vi "Periodic Tasks.vi"(8 "error in":errorcluster) -> ()   [LabVIEW 2015]
doc: "This VI runs in parallel to other tasks. It can contain as many user-defined periodic loops as you need. These can carry out PID or other sorts of timed response."
uses:
  <vilib>/Rock Robotics/WPI/Solenoid/WPI_SolenoidValue.ctl
  <vilib>/Rock Robotics/WPI/Utilities/WPI_GetSetVariantRefNum.vi
  <vilib>/Rock Robotics/WPI/Solenoid/WPI_SolenoidSetEnum.vi
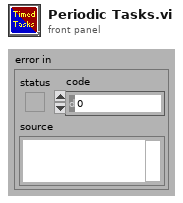
[diagram p1: front panel]
types:
  T1 = typedef "WPI_RobotDriveDevRef.ctl" = cluster{"DevStatus":errorcluster, "Motors[]":T2[], "Square Inputs":bool, "Max Output":dbl}
  T2 = typedef "WPI_MotorControlDeviceRef.ctl" = cluster{"DeviceStatus":errorcluster, "Type":T3, "PWM":cluster{"PWM Channel":T4, "DeadBand":T5}, "CAN":cluster{"Device Number":u8, "Control Mode":T6, "Semaphore":T7, "Max Vout":dbl, "TalonSRX Control Mode":T8}, "Invert":bool}
  T3 = typedef "WPI_MotorControlType.ctl" = enum16{"PWM", "CAN", "CANTalonSRX"}
  T4 = typedef "FPGA_DIOPWMChannel.ctl" = enum8{"PWM 0", "PWM 1", "PWM 2", "PWM 3", "PWM 4", "PWM 5", "PWM 6", "PWM 7", "PWM 8", "PWM 9", "PWM MXP 0", "PWM MXP 1", "PWM MXP 2", "PWM MXP 3", "PWM MXP 4", "PWM MXP 5", "PWM MXP 6", "PWM MXP 7", "PWM MXP 8", "PWM MXP 9", "Invalid"}
  T5 = typedef "WPI_PWMDeadband.ctl" = cluster{"Name":string, "maxPositivePwm":i32, "minPositivePwm":i32, "centerPwm":i32, "maxNegativePwm":i32, "minNegativePwm":i32, "angularRange":u16}
  T6 = typedef "WPI_CANJaguar_ControlMode.ctl" = enum8{"Percent VBus", "Current", "Speed", "Position", "Voltage"}
  T7 = typedef "Semaphore RefNum" = refnum<k1>
  T8 = typedef "WPI_CANTalonSRX_APIControlMode.ctl" = enum8{"Percent VBus", "Speed", "Position", "Slave", "Unchanged / Invalid", "Voltage Compensation", "Current", "Motion Profile"}
  T9 = typedef "WPI_JoystickDevRef.ctl" = cluster{"Device":T10}
  T10 = typedef "WPI_JoystickDeviceEnum.ctl" = enum16{"USB 0", "USB 1", "USB 2", "USB 3", "USB 4", "USB 5"}
  T11 = typedef "WPI_SolenoidDevRef.ctl" = cluster{"DevStatus":errorcluster, "Pneumatics Control Module":u8, "Forward Solenoid Channel":T12, "Reverse Solenoid Channel":T12}
  T12 = typedef "WPI_SolenoidChannel.ctl" = enum8{"Solenoid 0", "Solenoid 1", "Solenoid 2", "Solenoid 3", "Solenoid 4", "Solenoid 5", "Solenoid 6", "Solenoid 7", "Invalid"}
  T13 = cluster{"JoystickDevRef":T9, "RobotDriveDevRef":T1, "SolenoidDevRef":T11, "MotorControlDevRef":T2, "MotorControlDevRef":T2}
  T14 = typedef "WPI_SolenoidValue.ctl" = enum16{"Off", "On", "Forward", "Reverse"}
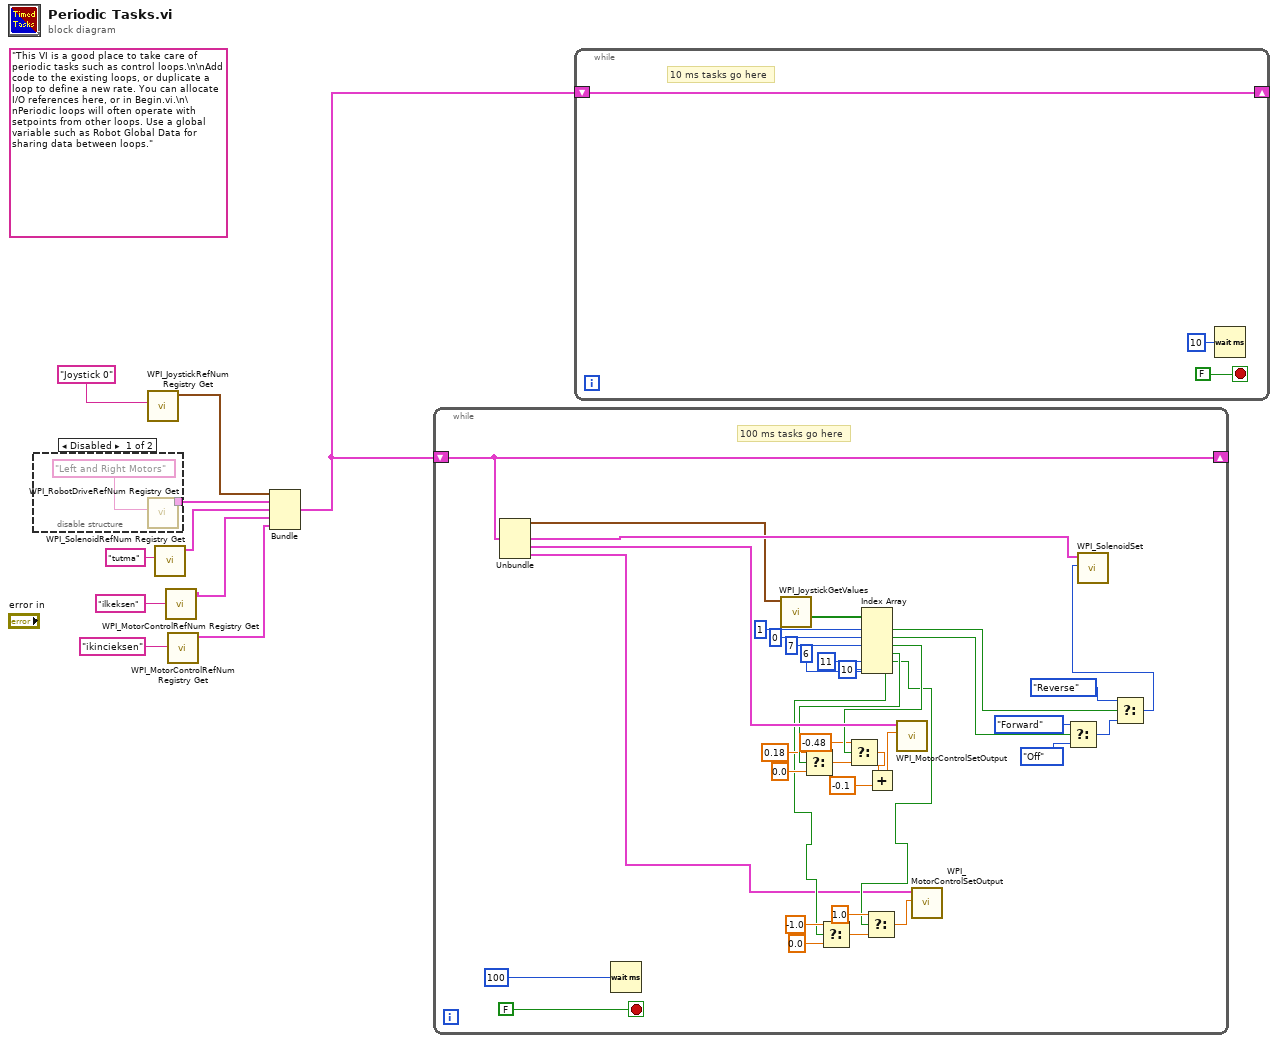
[diagram p0: block diagram]
diagram:
  (unwired) "This VI is a good place to take care of periodic tasks such as control loops.\n\nAdd code to the existing loops, or duplicate a loop to define a new rate. You can allocate I/O references here, or in Begin.vi.\n\nPeriodic loops will often operate with setpoints from other loops. Use a global variable such as Robot Global Data for sharing data between loops."
  n1 = disable-structure shown="Disabled" {
    disable-tunnel: [w11 _] -> w8
    frame Disabled {
      n2 = call <vilib>:"WPI_RobotDriveRefNum Registry Get.vi"("refnum name"="Left and Right Motors") -> ("RobotDriveDevRef"=w11:T1)  [unwired: 1 in, 9 out]
    }
    frame Enabled {
    }
  }
  n3 = call <vilib>:"WPI_JoystickRefNum Registry Get.vi"("refnum name"="Joystick 0") -> ("JoystickDevRef"=w9:T9)  [unwired: 1 in, 9 out]
  n4 = call <vilib>:"WPI_SolenoidRefNum Registry Get.vi"("refnum name"="tutma") -> ("SolenoidDevRef"=w5:T11)  [unwired: 9 in, 1 out]
  n5 = call <vilib>:"WPI_MotorControlRefNum Registry Get.vi"("refnum name"="ilkeksen") -> ("MotorControlDevRef"=w3:T2)  [unwired: 9 in, 1 out]
  n6 = call <vilib>:"WPI_MotorControlRefNum Registry Get.vi"("refnum name"="ikincieksen") -> ("MotorControlDevRef"=w1:T2)  [unwired: 9 in, 1 out]
  n7 = Bundle("JoystickDevRef"=w9, "RobotDriveDevRef"=w8, "SolenoidDevRef"=w5, "MotorControlDevRef"=w3, "MotorControlDevRef"=w1) -> (w7:T13)  [unwired: 1 out]
  n8 = while {
    shift-right: [w44] -> _
    shift-left: w7 -> [w44]
    stop <- FALSE stop-if-true
    # "100 ms tasks go here"
    n9 = Unbundle(w44) -> ("JoystickDevRef"=w42:T9, "SolenoidDevRef"=w43:T11, "MotorControlDevRef"=w41:T2, "MotorControlDevRef"=w16:T2)  [unwired: 1 out]
    n10 = Wait (ms)(milliseconds to wait=u32 100) -> ()  [unwired: 1 out]
    n11 = call <vilib>:"WPI_JoystickGetValues.vi"("JoystickDevRef"=w42) -> ("Buttons"=w45:bool[])  [unwired: 6 in, 4 out]
    n12 = Index Array "Index Array"(array=w45, index #1=1 ("index"), index #2=0 ("index"), index #3=7 ("index"), index #4=6 ("index"), index #5=11 ("index"), index #6=10 ("index")) -> (element #1=w26:bool, element #2=w25:bool, element #3=w38:bool, element #4=w36:bool, element #5=w17:bool, element #6=w18:bool)
    n13 = Select(t=0.18, s=w36, f=0.0) -> (s? t:f=w37:dbl)
    n14 = Select(t=-1.0, s=w18, f=0.0) -> (s? t:f=w23:dbl)
    n15 = Select(t=-0.48, s=w38, f=w37) -> (s? t:f=w13:dbl)
    n16 = Select(t=1.0, s=w17, f=w23) -> (s? t:f=w20:dbl)
    n17 = Add(x=w13, y=-0.1) -> (x+y=w14:dbl)
    n18 = call <vilib>:"WPI_MotorControlSetOutput.vi"("Output"=w14, "MotorControlDevRef"=w41) -> ()  [unwired: 7 in, 3 out]
    n19 = call <vilib>:"WPI_MotorControlSetOutput.vi"("Output"=w20, "MotorControlDevRef"=w16) -> ()  [unwired: 7 in, 3 out]
    n20 = Select(t=WPI_SolenoidValue."Forward" ("Value"), s=w25, f=WPI_SolenoidValue."Off") -> (s? t:f=w28:T14)
    n21 = Select(t=WPI_SolenoidValue."Reverse" ("Value"), s=w26, f=w28) -> (s? t:f=w24:T14)
    n22 = call-poly <vilib>:"WPI_SolenoidSet.vi"("Value"=w24, "SolenoidDevRef"=w43) -> ()  [unwired: 8 in, 2 out]
  }
  n23 = while {
    shift-right: [w50] -> _
    shift-left: w7 -> [w50]
    stop <- FALSE stop-if-true
    # "10 ms tasks go here"
    n24 = Wait (ms)(milliseconds to wait=u32 10) -> ()  [unwired: 1 out]
  }
